vi "Visa Write V2.vi"() -> ()   [LabVIEW 2022 SP3]
uses:
  <instrlib>/Keithley 2182/Keithley 2182.lvlib
panel:
  in  "2182A":T1={"Baud Rate"=9600, "Parity"=0, "Data Bits"=8, "Stop Bits"=10, "Flow Control"=0, "VISA resource name"="SourceMeter2400"} {"Flow Control" items=["None", "XON/XOFF", "RTS/CTS", "XON/XOFF & RTS/CTS", "DTR/DSR", "XON/XOFF & DTR/DSR"]; "Stop Bits" items=["1.0"=10, "1.5"=15, "2.0"=20]; "Data Bits" items=["7"=7, "8"=8]; "Parity" items=["None", "Odd", "Even", "Mark", "Space"]; "Baud Rate" items=["300"=300, "600"=600, "1200"=1200, "2400"=2400, "4800"=4800, "9600"=9600, "19200"=19200]}
  in  "2400":T1={"Baud Rate"=9600, "Parity"=0, "Data Bits"=8, "Stop Bits"=10, "Flow Control"=0, "VISA resource name"="SourceMeter2400"} {"Flow Control" items=["None", "XON/XOFF", "RTS/CTS", "XON/XOFF & RTS/CTS", "DTR/DSR", "XON/XOFF & DTR/DSR"]; "Stop Bits" items=["1.0"=10, "1.5"=15, "2.0"=20]; "Data Bits" items=["7"=7, "8"=8]; "Parity" items=["None", "Odd", "Even", "Mark", "Space"]; "Baud Rate" items=["300"=300, "600"=600, "1200"=1200, "2400"=2400, "4800"=4800, "9600"=9600, "19200"=19200]}
  out "Delta Readings (uV)":ext[](array[numeric]) format="%.12f"
  out "Voltage Drop Across DUT":dbl[](graph)
  in  "Sample Count To Display":i32=10
  out "Resistance (m-Ohms)":dbl[](array[numeric]) format="%.10f"
  out "Resistance of DUT":dbl[](graph)
  in  "2400 CURR LIST":string="20E-6,-20E-6"
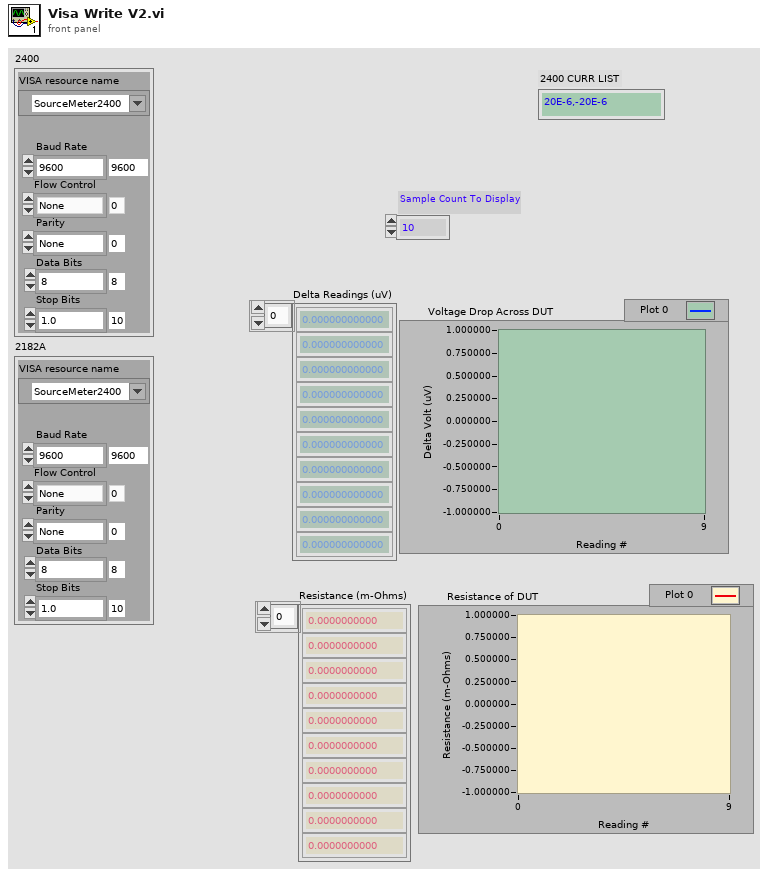
[diagram p1: front panel]
types:
  T1 = cluster{"Baud Rate":u32, "Parity":u16, "Data Bits":u16, "Stop Bits":u16, "Flow Control":u16, "VISA resource name":refnum<visa-resource-name>}
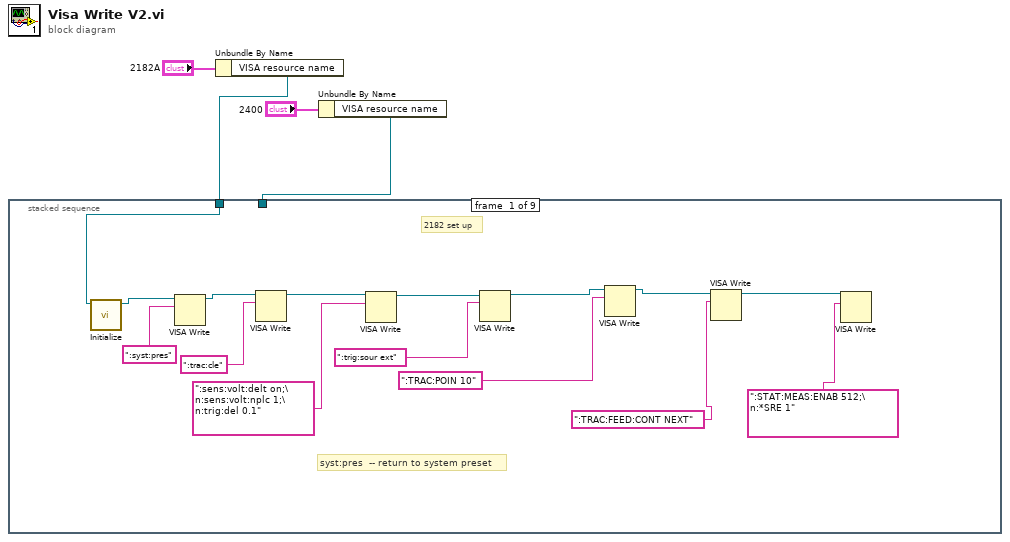
[diagram p0: block diagram]
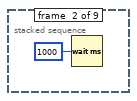
[diagram p2: hidden frame]
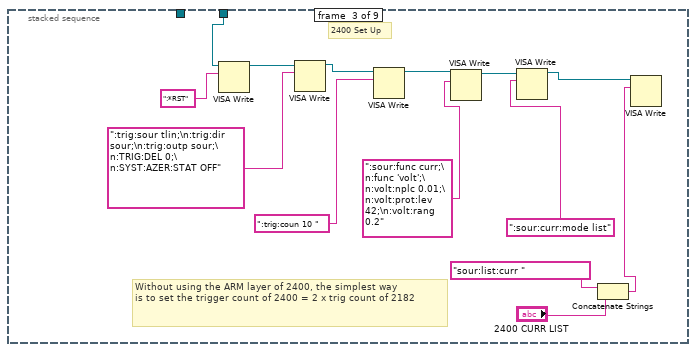
[diagram p3: hidden frame]
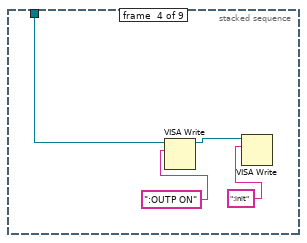
[diagram p4: hidden frame]
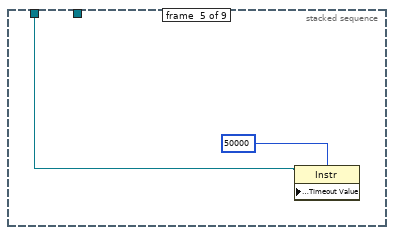
[diagram p5: hidden frame]
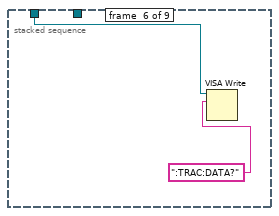
[diagram p6: hidden frame]
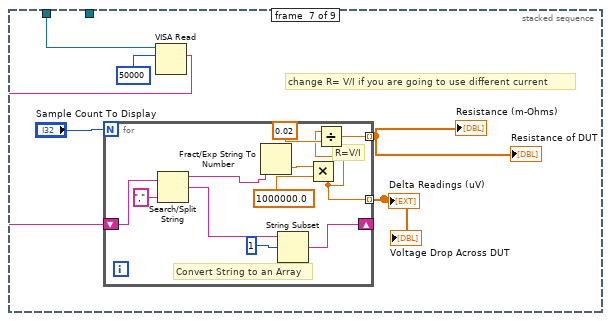
[diagram p7: hidden frame]
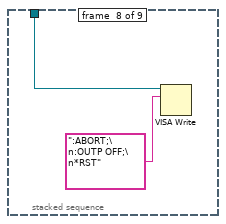
[diagram p8: hidden frame]
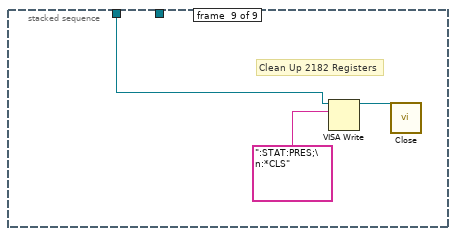
[diagram p9: hidden frame]
diagram:
  n1 = Unbundle By Name("2182A") -> ("VISA resource name"=w1:refnum<visa-resource-name>)
  n2 = Unbundle By Name("2400") -> ("VISA resource name"=w2:refnum<visa-resource-name>)
  n3 = stacked-sequence {
    tunnel: w1 -> [w6 _ _ _ w39 w41 w43 _ w63]
    tunnel: w2 -> [_ _ w32 w38 _ _ _ w61 _]
    frame #0 {
      # "syst:pres  -- return to system preset"
      # "2182 set up"
      n4 = call <instrlib>:"Initialize.vi"("VISA resource name"=w6) -> ("VISA resource name out"=w5:refnum<visa-resource-name>)  [unwired: 9 in, 1 out]
      n5 = VISA Write(VISA resource name=w5, write buffer=":syst:pres") -> (VISA resource name out=w7:refnum<visa-resource-name>)  [unwired: 1 in, 2 out]
      n6 = VISA Write(VISA resource name=w7, write buffer=":trac:cle") -> (VISA resource name out=w12:refnum<visa-resource-name>)  [unwired: 1 in, 2 out]
      n7 = VISA Write(VISA resource name=w12, write buffer=":sens:volt:delt on;\n:sens:volt:nplc 1;\n:trig:del 0.1") -> (VISA resource name out=w11:refnum<visa-resource-name>)  [unwired: 1 in, 2 out]
      n8 = VISA Write(VISA resource name=w11, write buffer=":trig:sour ext") -> (VISA resource name out=w10:refnum<visa-resource-name>)  [unwired: 1 in, 2 out]
      n9 = VISA Write(VISA resource name=w10, write buffer=":TRAC:POIN 10") -> (VISA resource name out=w9:refnum<visa-resource-name>)  [unwired: 1 in, 2 out]
      n10 = VISA Write(VISA resource name=w9, write buffer=":TRAC:FEED:CONT NEXT") -> (VISA resource name out=w8:refnum<visa-resource-name>)  [unwired: 1 in, 2 out]
      n11 = VISA Write(VISA resource name=w8, write buffer=":STAT:MEAS:ENAB 512;\n:*SRE 1") -> ()  [unwired: 1 in, 3 out]
    }
    frame #1 {
      n12 = Wait (ms)(milliseconds to wait=u32 1000) -> ()  [unwired: 1 out]
    }
    frame #2 {
      # "Without using the ARM layer of 2400, the simplest way\nis to set the trigger count of 2400 = 2 x trig count of 2182"
      # "2400 Set Up"
      n13 = VISA Write(VISA resource name=w32, write buffer=":*RST") -> (VISA resource name out=w31:refnum<visa-resource-name>)  [unwired: 1 in, 2 out]
      n14 = VISA Write(VISA resource name=w31, write buffer=":trig:sour tlin;\n:trig:dir sour;\n:trig:outp sour;\n:TRIG:DEL 0;\n:SYST:AZER:STAT OFF") -> (VISA resource name out=w30:refnum<visa-resource-name>)  [unwired: 1 in, 2 out]
      n15 = VISA Write(VISA resource name=w30, write buffer=":trig:coun 10 ") -> (VISA resource name out=w29:refnum<visa-resource-name>)  [unwired: 1 in, 2 out]
      n16 = VISA Write(VISA resource name=w29, write buffer=":sour:func curr;\n:func 'volt';\n:volt:nplc 0.01;\n:volt:prot:lev 42;\n:volt:rang 0.2") -> (VISA resource name out=w28:refnum<visa-resource-name>)  [unwired: 1 in, 2 out]
      n17 = VISA Write(VISA resource name=w28, write buffer=":sour:curr:mode list") -> (VISA resource name out=w27:refnum<visa-resource-name>)  [unwired: 1 in, 2 out]
      n18 = Concatenate Strings("sour:list:curr ", "2400 CURR LIST") -> (w21:string)
      n19 = VISA Write(VISA resource name=w27, write buffer=w21) -> ()  [unwired: 1 in, 3 out]
    }
    frame #3 {
      n20 = VISA Write(VISA resource name=w38, write buffer=":OUTP ON") -> (VISA resource name out=w37:refnum<visa-resource-name>)  [unwired: 1 in, 2 out]
      n21 = VISA Write(VISA resource name=w37, write buffer=":init") -> ()  [unwired: 1 in, 3 out]
    }
    frame #4 {
      n22 = property class="Instr"(reference=w39, "General Settings:Timeout Value"=u32 50000) -> ()  [unwired: 1 in, 2 out]
    }
    frame #5 {
      n23 = VISA Write(VISA resource name=w41, write buffer=":TRAC:DATA?") -> ()  [unwired: 1 in, 3 out]
    }
    frame #6 {
      # "change R= V/I if you are going to use different current"
      n24 = VISA Read(VISA resource name=w43, byte count=50000) -> (read buffer=w44:string)  [unwired: 1 in, 3 out]
      n25 = for {
        N: "Sample Count To Display" -> [_]
        tunnel: [w50] -> w47 mode=indexing
        shift-right: [w55] -> _
        shift-left: w44 -> [w56]
        tunnel: [w52] -> w46 mode=indexing
        # "R=V/I"
        # "Convert String to an Array"
        n26 = Search/Split String(string=w56, search string/char (-)=",") -> (substring before match=w58:string, match + rest of string=w57:string)  [unwired: 1 in, 1 out]
        n27 = Fract/Exp String To Number(string=w58) -> (number=w49:dbl)  [unwired: 3 in, 1 out]
        n28 = String Subset(string=w57, offset (0)=1) -> (substring=w55:string)  [unwired: 1 in]
        n29 = Multiply(x=w49, y=1000000.0) -> (x*y=w50:dbl)
        n30 = Divide(x=w50, y=0.02 ("x")) -> (x/y=w52:dbl)
      }
      "Delta Readings (uV)" <- w47
      "Voltage Drop Across DUT" <- w47
      "Resistance (m-Ohms)" <- w46
      "Resistance of DUT" <- w46
    }
    frame #7 {
      n31 = VISA Write(VISA resource name=w61, write buffer=":ABORT;\n:OUTP OFF;\n*RST" ("data")) -> ()  [unwired: 1 in, 3 out]
    }
    frame #8 {
      # "Clean Up 2182 Registers"
      n32 = VISA Write(VISA resource name=w63, write buffer=":STAT:PRES;\n:*CLS" ("data")) -> (VISA resource name out=w62:refnum<visa-resource-name>)  [unwired: 1 in, 2 out]
      n33 = call <instrlib>:"Close.vi"("VISA resource name"=w62) -> ()  [unwired: 10 in, 1 out]
    }
  }
